vi "Synchronize to GPS - cRIO.vi"() -> ()   [LabVIEW 2011]
uses:
  <vilib>/rvi/eio/common/nirviEmuTemplateMethod_errors.vi
  <vilib>/rvi/eio/common/nirviEmuTemplatePropertyGet_noerrors.vi
  <vilib>/eio/EIOMethodNode/EIOMethodNode.xnode
  <vilib>/eio/EIOPropertyNode/EIOPropertyNode.xnode
  FPGA Timekeeper.lvlib
  <vilib>/rvi/eio/common/nirviEmuTemplatePropertyGet_errors.vi
  <vilib>/rvi/eio/common/nirviEmuTemplatePropertySet_errors.vi
  <vilib>/rvi/eio/common/nirviEmuTemplatePropertySet_noerrors.vi
panel:
  out "UTC offset valid":bool
  out "UTC offset":i8
  out "satellites available":u8
  out "antenna status":T1(ring)
  out "GPS status":T2(ring)
  out "offset from time reference":i32
  out "FPGA Timekeeper locked":bool
  out "FPGA Timekeeper time (ns)":u64
  # "This example synchronizes the FPGA Timekeeper on a CompactRIO FPGA target with a GPS pulse per second (PPS)."
  # "GPS"
  # "FPGA Timekeeper"
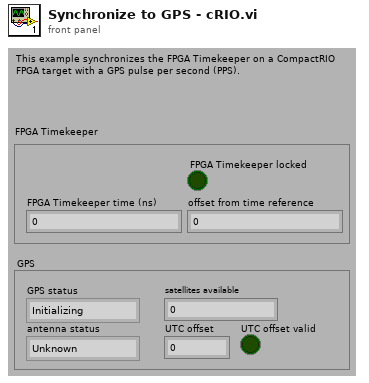
[diagram p1: front panel]
types:
  T1 = enum8{"Unknown", "Normal", "Absent", "Overcurrent"}
  T2 = enum8{"Initializing", "Normal", "Unable to get fix"}
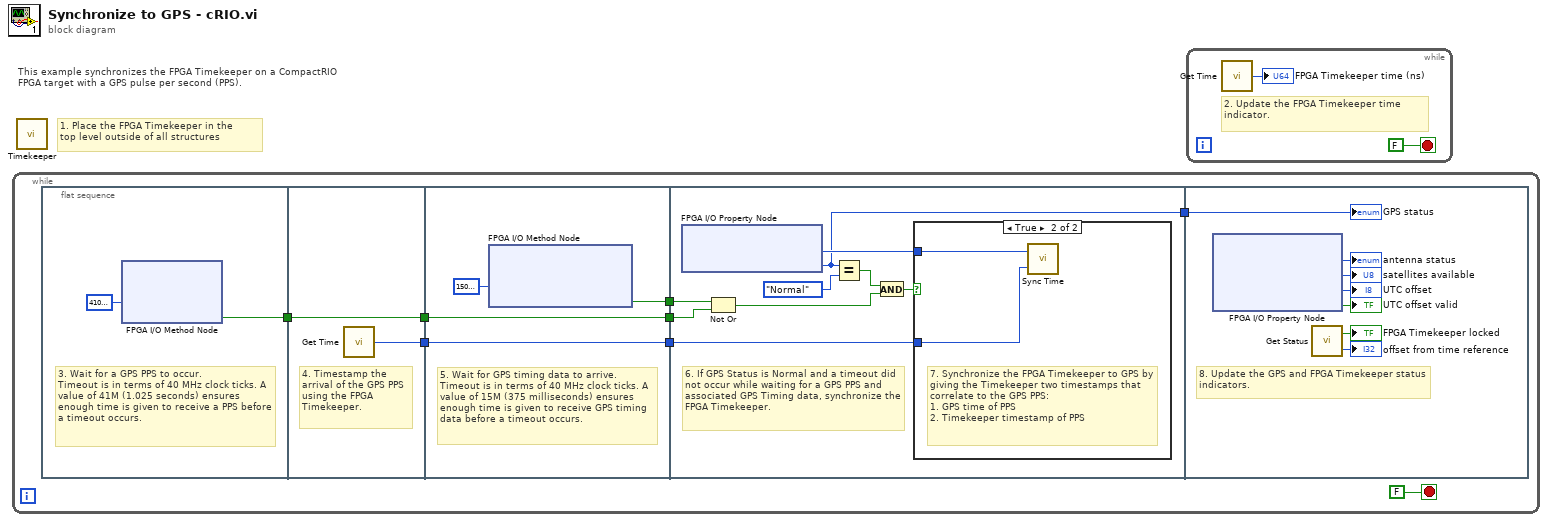
[diagram p0: block diagram]
diagram:
  # "This example synchronizes the FPGA Timekeeper on a CompactRIO FPGA target with a GPS pulse per second (PPS)."
  # "1. Place the FPGA Timekeeper in the\ntop level outside of all structures"
  n1 = while {
    stop <- FALSE stop-if-true
    n2 = flat-sequence {
      tunnel: [w9] -> w7
      tunnel: w7 -> [w12]
      tunnel: [w12] -> w6
      tunnel: [w11] -> w4
      tunnel: [w15] -> w8
      tunnel: w6 -> [w14]
      tunnel: [w14] -> w5
      tunnel: w4 -> [w13]
      tunnel: [w13] -> w3
      tunnel: w8 -> [w24]
      tunnel: w5 -> [w23]
      tunnel: w3 -> [w18]
      tunnel: [w17] -> w2
      tunnel: w2 -> [w34]
      frame #0 {
        # "3. Wait for a GPS PPS to occur.\nTimeout is in terms of 40 MHz clock ticks. A value of 41M (1.025 seconds) ensures enough time is given to receive a PPS before a timeout occurs."
        n3 = xnode "FPGA I/O Method Node"("Timeout"=41000000) -> ("Timed Out"=w9:bool)  [unwired: 1 in, 1 out]
      }
      frame #1 {
        # "4. Timestamp the arrival of the GPS PPS using the FPGA Timekeeper."
        n4 = call "Get Time.vi"() -> ("time (ns)"=w11:u64)
      }
      frame #2 {
        # "5. Wait for GPS timing data to arrive.\nTimeout is in terms of 40 MHz clock ticks. A value of 15M (375 milliseconds) ensures enough time is given to receive GPS timing data before a timeout occurs."
        n5 = xnode "FPGA I/O Method Node"("Timeout"=15000000) -> ("Timed Out"=w15:bool)  [unwired: 1 in, 1 out]
      }
      frame #3 {
        # "6. If GPS Status is Normal and a timeout did not occur while waiting for a GPS PPS and associated GPS Timing data, synchronize the FPGA Timekeeper."
        n6 = xnode "FPGA I/O Property Node"() -> ("PPS Timestamp (TAI)"=w19:u64, "GPS Status"=w17:T2)  [unwired: 1 in, 1 out]
        n7 = Not Or(1:w23, 2:w24) -> (0:w21:bool)
        n8 = Equal?(x=w17, y=T2."Normal") -> (x = y?=w22:bool)
        n9 = And(x=w22, y=w21) -> (x .and. y?=w20:bool)
        n10 = case shown="True" w20 {
          tunnel: w19 -> [_ w27]
          tunnel: w18 -> [_ w26]
          frame False {
          }
          frame True {
            # "7. Synchronize the FPGA Timekeeper to GPS by giving the Timekeeper two timestamps that correlate to the GPS PPS:\n1. GPS time of PPS\n2. Timekeeper timestamp of PPS"
            n11 = call "Sync Time.vi"("FPGA Timekeeper time (ns)"=w26, "time reference time (ns)"=w27) -> ()
          }
        }
      }
      frame #4 {
        # "8. Update the GPS and FPGA Timekeeper status indicators."
        n12 = xnode "FPGA I/O Property Node"() -> ("Antenna Status"=→"antenna status":T1, "Satellites Available"=→"satellites available":u8, "UTC Offset"=→"UTC offset":i8, "UTC Offset Valid"=→"UTC offset valid":bool)  [unwired: 1 in, 1 out]
        n13 = call "Get Status.vi"() -> ("FPGA Timekeeper locked"=→"FPGA Timekeeper locked":bool, "offset from time reference"=→"offset from time reference":i32)
        "GPS status" <- w34
      }
    }
  }
  n14 = call "Timekeeper.vi"() -> ()  [unwired: 12 in]
  n15 = while {
    stop <- FALSE stop-if-true
    # "2. Update the FPGA Timekeeper time indicator."
    n16 = call "Get Time.vi"() -> ("time (ns)"=→"FPGA Timekeeper time (ns)":u64)
  }
